vi "Results Display Updater.vi"(10 "Array of Results Reference":refnum<vi>, 11 "New Results":T1 {"Percentage Error Rates" format="%.1f%%"; "Test Frequency" format="%.0f MHz"}) -> ()   [LabVIEW 2013]
doc: "This VI updates the 'live results' window on the UI by reference."
uses:
  Test Results Display Cluster.ctl
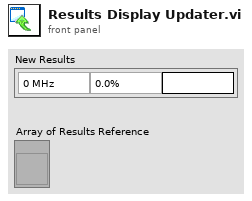
[diagram p1: front panel]
types:
  T1 = typedef "Test Results Display Cluster.ctl" = cluster{"Test Frequency":u32, "Percentage Error Rates":dbl, "Results":string}
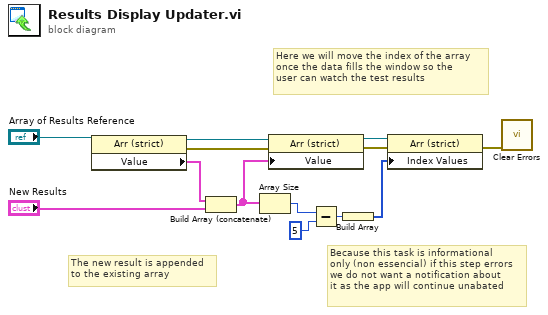
[diagram p0: block diagram]
diagram:
  # "Because this task is informational\nonly (non essencial) if this step errors\nwe do not want a notification about\nit as the app will continue unabated"
  # "The new result is appended\nto the existing array"
  # "Here we will move the index of the array\nonce the data fills the window so the\nuser can watch the test results"
  n1 = property class="Arr (strict)"(reference="Array of Results Reference") -> (reference out=w12:refnum<vi>, error out=w9:errorcluster, "Value"=w10:T1[])  [unwired: 1 in]
  n2 = Build Array (concatenate)(w10, "New Results") -> (w6:T1[])
  n3 = Array Size(array=w6) -> (size(s)=w5:i32)
  n4 = property class="Arr (strict)"(reference=w12, error in=w9, "Value"=w6) -> (reference out=w8:refnum<vi>, error out=w7:errorcluster)
  n5 = Subtract(x=w5, y=5) -> (x-y=w3:i32)
  n6 = Build Array(w3) -> (w2:i32[])
  n7 = property class="Arr (strict)"(reference=w8, error in=w7, "Index Values"=w2) -> (error out=w1:errorcluster)  [unwired: 1 out]
  n8 = call <vilib>:"Clear Errors.vi"("error in (no error)"=w1) -> ()  [unwired: 6 in, 1 out]
